vi "Get DataRead.vi"(8 "error in (no error)":errorcluster caption="entrée d'erreur (pas d'erreur)", 11 "Server TCP_IP P2110 en entrée":refnum<class "Server TCP_IP P2110.lvclass">) -> (0 "error out":errorcluster caption="sortie d'erreur", 2 "DataRead":T1, 3 "Server TCP_IP P2110 en sortie":refnum<class "Server TCP_IP P2110.lvclass">)   [LabVIEW 2020, in "Library Instrument & Equipement.lvlib" / "Library TCP IP.lvlib" / "Server TCP_IP P2110.lvclass"]
uses:
  Server TCP_IP P2110.lvclass
  C:/Users/ngarcin/OneDrive - Altyor/Standard TB/Class/TCP IP/Server TCP_IP (Default)/Server TCP_IP (Default).lvclass
  Server TCP_IP P2110.lvclass/Server TCP_IP P2110.ctl
  JSON API/JSON Value/Set from JSON string.vi
  JSON API/JSON Value/JSON Value.lvclass
  JSON API/Variant JSON/Variant JSON.lvlib
  JSON API/Get Polymorphic/JSON GetSet.lvlib
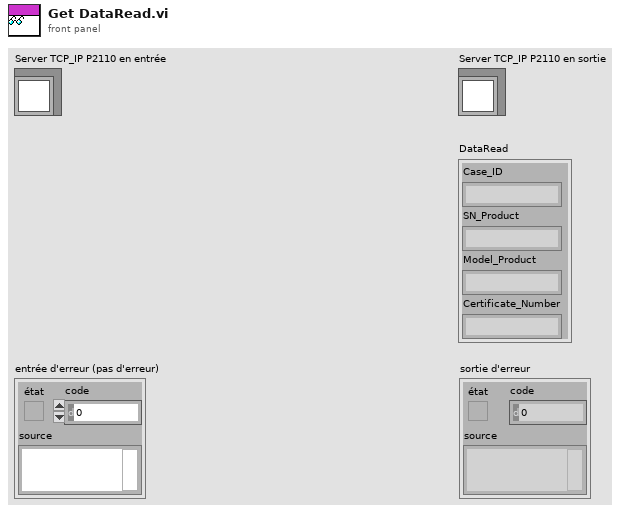
[diagram p1: front panel]
types:
  T1 = cluster{"Case_ID":string, "SN_Product":string, "Model_Product":string, "Certificate_Number":string}
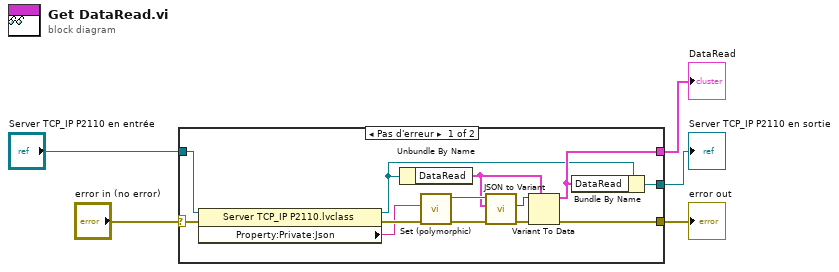
[diagram p0: block diagram]
diagram:
  n1 = case shown="Pas d'erreur" "error in (no error)" {
    selector: "error in (no error)" -> [w7 w19]
    tunnel: [w6 w19] -> w4
    tunnel: [w8 w20] -> w2
    tunnel: "Server TCP_IP P2110 en entrée" -> [w13 w20]
    tunnel: [w10 _] -> w1
    frame No Error {
      n2 = property class="Server TCP_IP P2110.lvclass"(reference=w13, error in=w7) -> (reference out=w9:refnum<class "Server TCP_IP P2110.lvclass">, error out=w14:errorcluster, "Property:Private:Json"=w12:string)
      n3 = Unbundle By Name(w9) -> ("DataRead"=w11:T1)
      n4 = call-poly "Set (polymorphic).vi"("error in (no error)"=w14, "JSON stream"=w12) -> ("error out"=w16:errorcluster, "JSON Value out"=w18:refnum<class "JSON Value.lvclass">)  [unwired: 7 in, 1 out]
      n5 = call "JSON to Variant.vi"("error in (no error)"=w16, "Variant (Data Type)"=w11, "JSON Value"=w18) -> ("error out"=w17:errorcluster, "Variant out"=w15:variant)  [unwired: 7 in]
      n6 = Variant To Data(error in=w17, type=w11, Variant=w15) -> (data=w10:T1, error out=w6:errorcluster)
      n7 = Bundle By Name(cluster=w9, "DataRead"=w10) -> (w8:refnum<class "Server TCP_IP P2110.lvclass">)
    }
    frame Error {
    }
  }
  "error out" <- w4
  "Server TCP_IP P2110 en sortie" <- w2
  "DataRead" <- w1
